vi "3.vi"() -> ()   [LabVIEW 2017]
panel:
  out "数组":i32[](array[numeric])
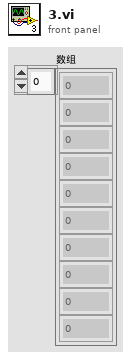
[diagram p1: front panel]
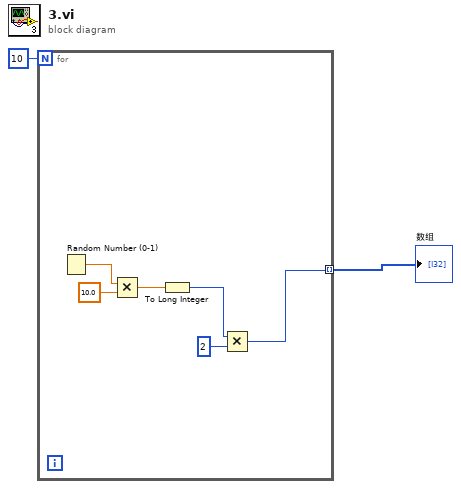
[diagram p0: block diagram]
diagram:
  n1 = for {
    N: 10 -> [_]
    tunnel: [w3] -> w1 mode=indexing
    n2 = Random Number (0-1)() -> (number: 0 to 1=w8:dbl)
    n3 = Multiply(x=w8, y=10.0) -> (x*y=w6:dbl)
    n4 = To Long Integer(number=w6) -> (32bit integer=w5:i32)
    n5 = Multiply(x=w5, y=2) -> (x*y=w3:i32)
  }
  "数组" <- w1
